vi "lookupService.vi"(3 "Err In":path, 5 "Service ROS":T2={"topic port"=0, "Node"="", "topic"="", "type"="", "node port"=0, "error "={"status"=FALSE, "code"=0, "source"=""}, "Direction"=enum."Node", "APIs"=[], "Update (ms)"=1, "write queue"=1}) -> (0 "Err Out":path, 1 "Log":T1)   [LabVIEW 2012]
uses:
  <userlib>/ROSforLV/ROS/Code/SubVIs/_ROSControl.ctl
  <userlib>/ROSforLV/ROS/Code/SubVIs/_ROSDirection.ctl
  <userlib>/ROSforLV/ROS/Code/Console/Servers/ServerSubs/ROSLog.ctl
  <userlib>/ROSforLV/ROS/Code/Console/Servers/ServerSubs/MyState.ctl
  <userlib>/ROSforLV/ROS/Code/_ROSDefinition.vi
panel:
  out "response":string
  out "lookupService":string="POST /RPC2 HTTP/1.1\r\nHost: 192.168.1.110:11311\r\nContent-Type: text/xml\r\nContent-Length: 396\r\n\r\n<?xml version='1.0'?>\n<methodCall>\r <methodName>registerSubscriber</methodName>\r <params>\r   <param><value><string>/ChrisAir</string> </value> </param>\r   <param><value><string>/robot/joint_states</string> </value> </param>\r   <param><value><string>sensor_msgs/JointState</string> </value> </param>\r   <param><value><string>http://192.168.1.111</string> </value> </param>\r </params>\r</methodCall>"
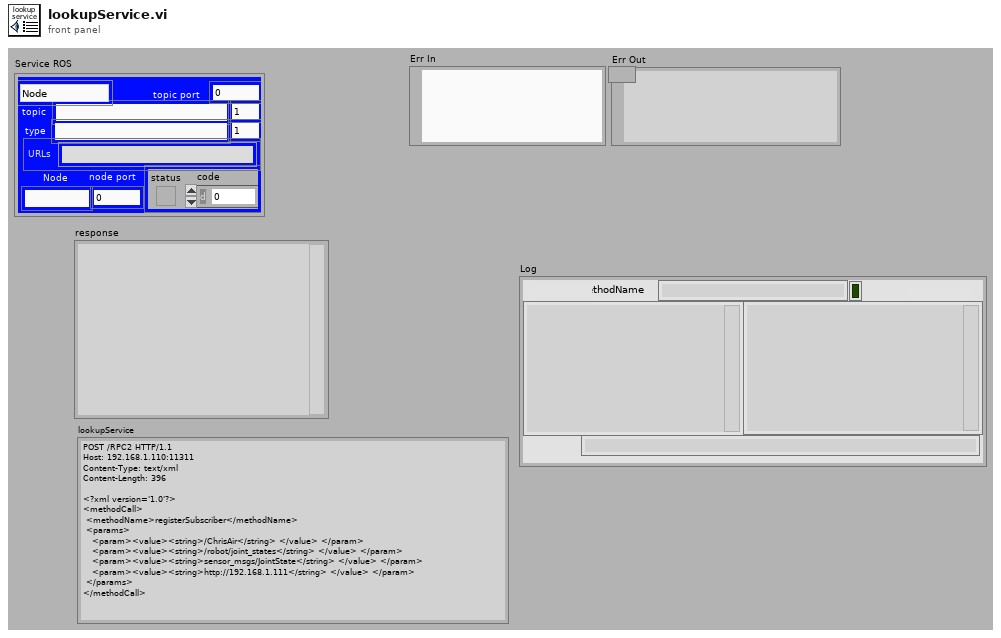
[diagram p1: front panel]
types:
  T1 = typedef "ROSLog.ctl" = cluster{"Sent":string, "Reply":string, "MethodName":string, "success":bool, "Dir1":string, "Dir2":string, "Time Stamp":string, "error":errorcluster, "Preamble":string}
  T2 = typedef "_ROSControl.ctl" = cluster{"topic port":u16, "Node":string, "topic":string, "type":string, "node port":u32, "error ":errorcluster, "Direction":T3, "APIs":string[], "Update (ms)":u16, "write queue":u16}
  T3 = typedef "_ROSDirection.ctl" = enum16{"Node", "Publisher", "Subscriber", "Service Client"}
  T4 = enum16{"Reset Log", "Add Client", "Remove Client", "Add Task"}
  T5 = typedef "MyState.ctl" = enum16{"No Connection", "Registered", "Connected", "Close"}
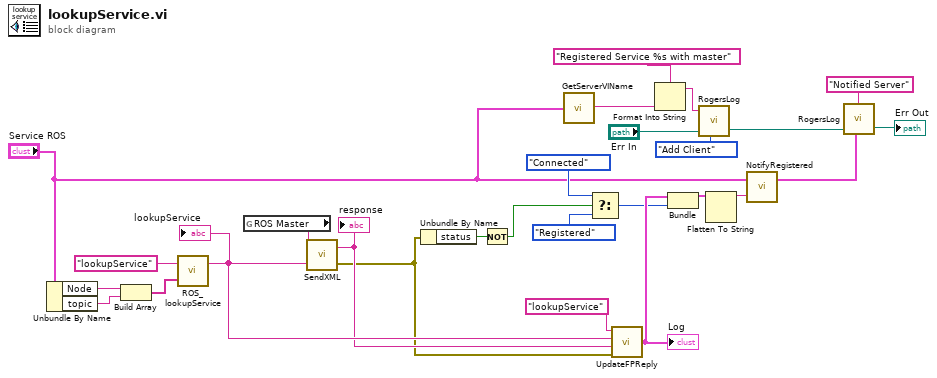
[diagram p0: block diagram]
diagram:
  n1 = Unbundle By Name("Service ROS") -> ("Node"=w27:string, "topic"=w26:string)
  n2 = Build Array(w27, w26) -> (w25:string[])
  n3 = call <userlib>:"ROS_lookupService.vi"("Parameters"=w25, "Method Name"="lookupService") -> ("lookupService"=w23:string)  [unwired: 1 in]
  "lookupService" <- w23
  n4 = global read "_ROSDefinition.vi" "ROS Master"() -> (w19:string)
  n5 = call <userlib>:"SendXML.vi"("Send"=w23, "URI in"=w19) -> ("error out"=w11:errorcluster, "Reply"=w22:string)
  "response" <- w22
  n6 = Unbundle By Name(w11) -> ("status"=w20:bool)
  n7 = Not(x=w20) -> (.not. x?=w15:bool)
  n8 = call <userlib>:"GetServerVIName.vi"("ROS"="Service ROS") -> ("vi name"=w3:string)
  n9 = Select(t=MyState."Connected" ("MyState"), s=w15, f=MyState."Registered" ("MyState")) -> (s? t:f=w12:T5)
  n10 = call <userlib>:"UpdateFPReply.vi"("error in (no error)"=w11, "Reply"=w22, "Sent"=w23, "method"="lookupService" ("Method Name")) -> ("Log"=w17:T1)
  "Log" <- w17
  n11 = Format Into String(format string="Registered Service %s with master" ("Text to add"), w3) -> (resulting string=w5:string)  [unwired: 2 in, 1 out]
  n12 = Bundle("Log"=w17, "MyState"=w12) -> (w16:cluster{"Log":T1, "MyState":T5})  [unwired: 1 in]
  n13 = call <userlib>:"RogersLog.vi"("Text to add"=w5, "LogPath in"="Err In", "Task"=T4."Add Client") -> ("LogPath out"=w8:path)  [unwired: 2 in, 1 out]
  n14 = Flatten To String(anything=w16) -> (data string=w18:string)  [unwired: 3 in, 2 out]
  n15 = call <userlib>:"NotifyRegistered.vi"("data string"=w18, "ROS"="Service ROS") -> ("ROS out"=w1:T2)  [unwired: 1 in]
  n16 = call <userlib>:"RogersLog.vi"("Text to add"="Notified Server", "ROS"=w1, "LogPath in"=w8) -> ("LogPath out"=→"Err Out":path)  [unwired: 2 in, 1 out]
